vi "Put_I64-1D_PV.vi"(5 "variable PV names (F)":bool, 7 "Synchronous (F)":bool, 8 "Error in (no error)":errorcluster, 9 "Timeout (3)":dbl=3.0, 10 "Values":i64[](array[numeric]), 11 "PV Name":string) -> (0 "Error out":errorcluster, 1 "PV error":errorcluster, 2 "Status":bool, 3 "PV Name (dup)":string)   [LabVIEW 2018]
doc: "This is a polymorphic VI for setting values of EPICS variables.\n\nINPUT:\n <b>PV name(s)</b>\n name of EPICS variable\n <b>value(s)</b>\n Boolean value OR Double value OR Double array OR String array\n <b>timeout</b>\n optional\n timeout for Channel Access requests\n <b>error in</b>\n <b>buffer size (since version 1.3 without function)</b>\n <b>synchronous</b>\n optional\n TRUE=synchronous; FALSE=asynchronous\n synchronous = writes value(s) after waiting for end of record processing\n <b>ValueSetsInColumns</b>\n optional\n TRUE = use columns for value sets instead of rows\n\nOUTPUT:\n <b>PV name(s)</b>\n name of EPICS variable\n </b>status</b>\n FALSE: request successful\n TRUE: warnings or errors\n <b>errors</b>\n resulting errors of all put commands\n <b>error out</b>\n global io error"
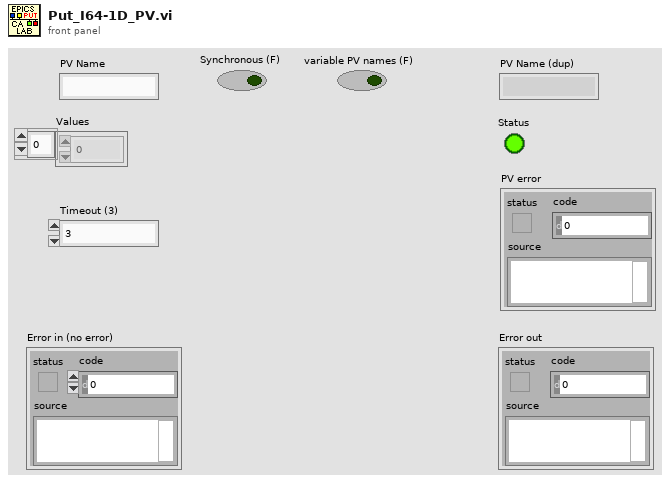
[diagram p1: front panel]
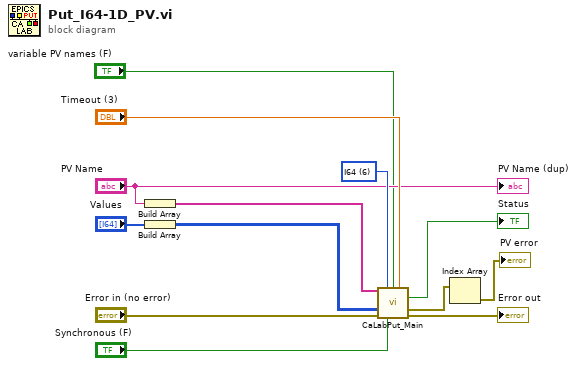
[diagram p0: block diagram]
diagram:
  w13 = 6 items=["String", "SGL", "DBL", "I8", "I16", "I32", "I64"] ("data type")
  n1 = Build Array("PV Name") -> (w5:string[])
  n2 = Build Array("Values") -> (w6:i64[][])
  n3 = call <userlib>:"CaLabPut_Main.vi"("PV Names"=w5, "Data Type"=w13, "variable PV names (F)"="variable PV names (F)", "Timeout (3)"="Timeout (3)", "Values [I64]"=w6, "Error in (no error)"="Error in (no error)", "Synchronous"="Synchronous (F)") -> ("Status"=→"Status":bool, "PV Errors"=w2:errorcluster[], "Error out"=→"Error out":errorcluster)  [unwired: 3 in, 3 out]
  n4 = Index Array(array=w2) -> (element=→"PV error":errorcluster)  [unwired: 1 in]
  "PV Name (dup)" <- "PV Name"
